vi "DoNotWaitOnTestComplete_Init.vi"(8 "error in (no error)":errorcluster, 10 "methodName (\"runTest\")":string="runTest", 11 "reference in":refnum<class "DoNotWaitOnTestComplete.lvclass">) -> (0 "error out":errorcluster, 3 "reference out":refnum<class "DoNotWaitOnTestComplete.lvclass">)   [LabVIEW 2011, in "DoNotWaitOnTestComplete.lvclass"]
uses:
  DoNotWaitOnTestComplete.lvclass
  DoNotWaitOnTestComplete.lvclass/DoNotWaitOnTestComplete.ctl
  Classes/TestCase/TestCase.lvclass
panel:
  # "Copyright © 2007 James Kring, Inc. All rights reserved.\n\nAuthor: Jim Kring [jim.kring@jameskring.com]\n\nThis library is provided \"AS IS\" ,WITHOUT WARRANTIES OR \nCONDITIONS OF ANY KIND, either express or implied.\n\nJames Kring, Inc. -- http://www.jameskring.com"
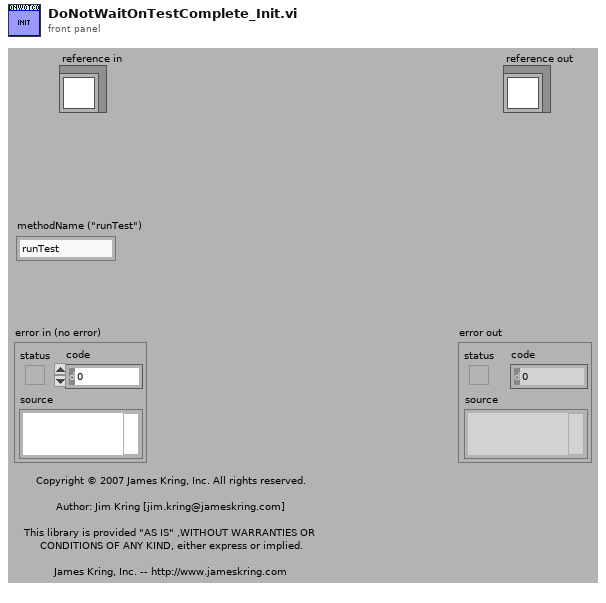
[diagram p1: front panel]
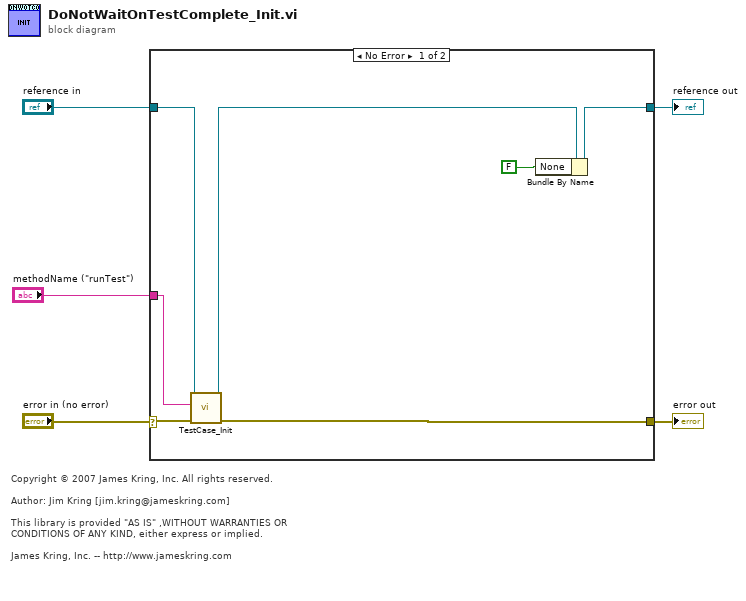
[diagram p0: block diagram]
diagram:
  # "Copyright © 2007 James Kring, Inc. All rights reserved.\n\nAuthor: Jim Kring [jim.kring@jameskring.com]\n\nThis library is provided \"AS IS\" ,WITHOUT WARRANTIES OR \nCONDITIONS OF ANY KIND, either express or implied.\n\nJames Kring, Inc. -- http://www.jameskring.com"
  n1 = case shown="No Error" "error in (no error)" {
    selector: "error in (no error)" -> [w10 w13]
    tunnel: [w12 w14] -> w5
    tunnel: "reference in" -> [w8 w14]
    tunnel: [w9 w13] -> w2
    tunnel: "methodName (\"runTest\")" -> [w6 _]
    frame No Error {
      n2 = call "TestCase_Init.vi"("error in (no error)"=w10, "methodName (\"runTest\")"=w6, "TestCase in"=w8) -> ("error out"=w9:errorcluster, "TestCase out"=w7:refnum<class "DoNotWaitOnTestComplete.lvclass">)  [unwired: 7 in]
      n3 = Bundle By Name(cluster=w7, "None"=FALSE) -> (w12:refnum<class "DoNotWaitOnTestComplete.lvclass">)
    }
    frame Error {
    }
  }
  "reference out" <- w5
  "error out" <- w2
